vi "ecg_ncs_v1.vi"() -> ()   [LabVIEW 2016]
uses:
  <instrlib>/niUSRP/niUSRP Timestamp.ctl
  C:/Program Files/National Instruments/LabVIEW 2016/examples/Instrument IO/Serial/support/Serial - Settings.ctl
  State.ctl
  <vilib>/Instr/_visa.llb/VISA Configure Serial Port (Instr).vi
  <instrlib>/niUSRP/niUSRP Write Tx Data (2D CDB).vi
  <instrlib>/niUSRP/niUSRP Fetch Rx Data (2D CDB).vi
panel:
  out "error IO 2":errorcluster={"status"=FALSE, "code"=-1074118647, "source"=""}
  in  "Serial Settings":T1={"baud rate"=57600, "data bits"=8, "parity"=enum."None", "stop bits"=10, "flow control"=0} {"flow control" items=["None"=0, "XON/XOFF"=1, "RTS/CTS"=2, "DTR/DSR"=4]; "stop bits" items=["1.0"=10, "1.5"=15, "2.0"=20]; "data bits" min=5 max=8 step=1; "baud rate" items=["75"=75, "110"=110, "134"=134, "150"=150, "300"=300, "600"=600, "1200"=1200, "1800"=1800, "2400"=2400, "4800"=4800, "7200"=7200, "9600"=9600, "14400"=14400, "19200"=19200, "28800"=28800, "38400"=38400, "56000"=56000, "57600"=57600, "115200"=115200, "128000"=128000, "230400"=230400]}
  in  "VISA resource name":refnum<visa-resource-name>="bmd101"
  out "Packets Recieved":i32
  out "ECG":i16(graph)
  in  "byte count":u32=1
  in  "Stop 2":bool
  out "Coerced Rx IQ Rate":dbl
  in  "Sampling Rate":i32=500
  out "Gain":dbl=-15.0
  out "Bandwidth":dbl=56000000.0
  out "Coerced Carrier Frequency":dbl=2000000000.0 format="%#.17g"
  out "Coerced Tx IQ rate":dbl=1000000.0
  out "error IO":errorcluster={"status"=FALSE, "code"=-1074118647, "source"=""}
  in  "Rx Number of Samples":i32=20000
  in  "Tab Control 2":enum32{"NI-294x/295x", "NI-2900/2901"}(tab)=enum."NI-2900/2901"
  in  "Rx carrier frequency [Hz]":dbl=2000000000.0 format="%#_6p"
  in  "Tx carrier frequency [Hz]":dbl=1000000000.0 format="%#_6p"
  in  "Start Trigger Time":T2={"whole seconds"=1, "fractional seconds"=0.0}
  in  "Tab Control":T3(tab)
  out "NCS tag Amp":dbl[](graph)=[0.011967714738528729, 0.012021355192189592, 0.012015275039596582, 0.011969166030167903, 0.011958890166168242, 0.012007893820858737, 0.012022893722444085, 0.011978222225113794, 0.011969989939463181, 0.012003099640895068]
  out "NCS tag Phase":dbl[](graph)=[0.011967714738528729, 0.012021355192189592, 0.012015275039596582, 0.011969166030167903, 0.011958890166168242, 0.012007893820858737, 0.012022893722444085, 0.011978222225113794, 0.011969989939463181, 0.012003099640895068]
  out "Tag Amp":dbl[](graph)
  out "Tag Phase":dbl[](graph)
  out "Tx Waveform Graph":waveform(dbl)[](graph)
  in  "Stop":bool
  in  "Channel 0\nTone Amplitude":dbl=0.707 step=0.05 format="%#.6g"
  in  "Channel 0 \nTone Frequency":dbl=5000.0 format="%#_6p"
  in  "Tx Waveform Size":dbl=2000.0
  in  "Device Name":refnum<k15>="MyB200"
  in  "Tx Gain":dbl=28.0 format="%#_6f"
  in  "Tx IQ Rate":dbl=1000000.0 format="%#_6p"
  in  "Rx Gain":dbl=32.0 format="%#_6f"
  in  "Rx IQ Rate":dbl=1000000.0 format="%#_6p"
  # "Rx Settings"
  # "Tx Settings"
  # "Note that on the NI-2900 and NI-2901, both Rx channels share an LO and both Tx channels share an LO. However, on the NI-294x/295x devices, Rx and Tx of channel 0 share an LO and Rx and Tx of channel 1 share an LO."
  # "This Tx graph should always have end and start tied up since this is being sent in a loop continuously. Otherwise phase jumps will be noticed."
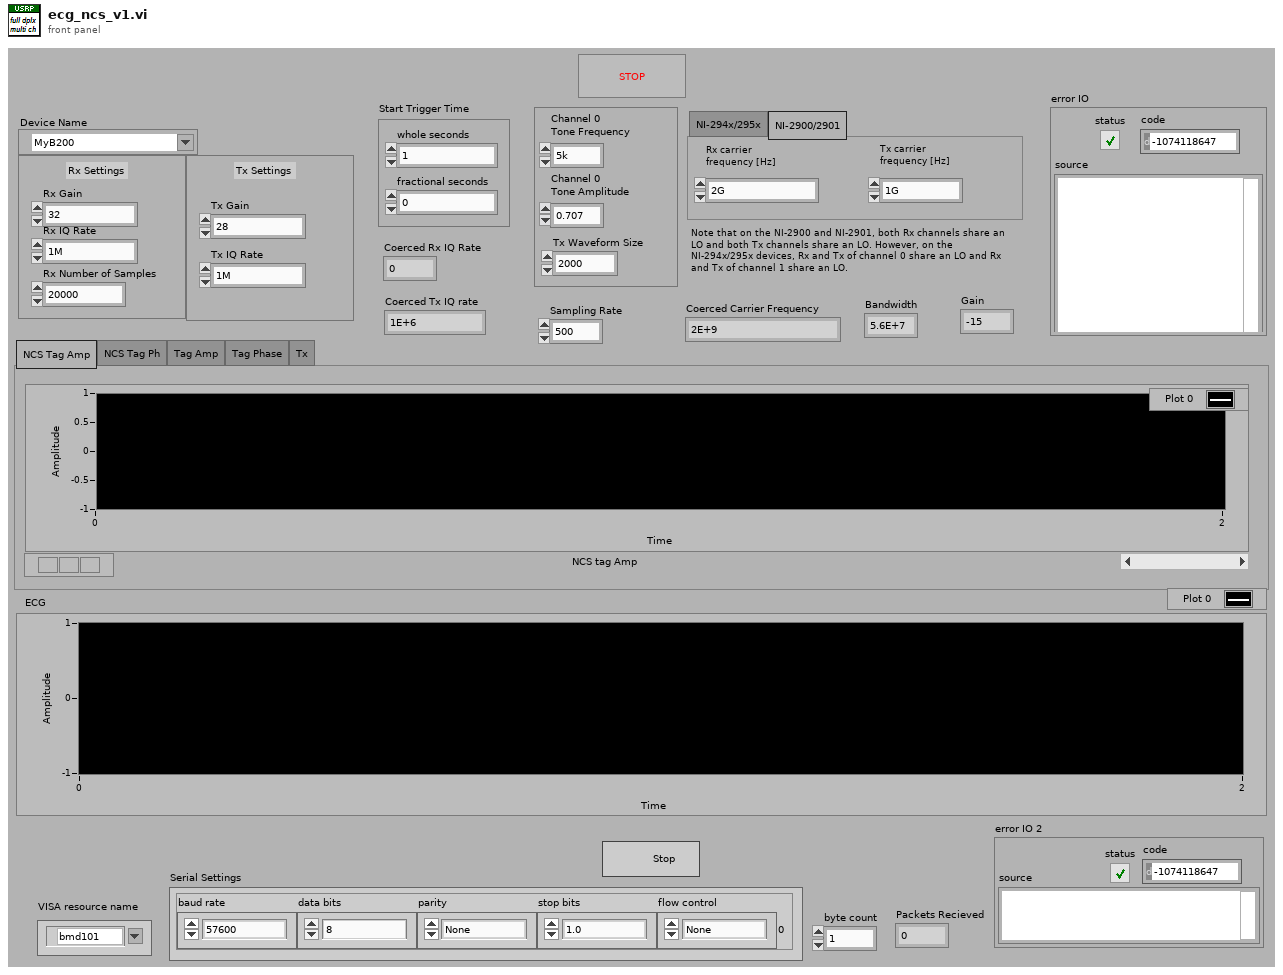
[diagram p1: front panel]
types:
  T1 = typedef "Serial - Settings.ctl" = cluster{"baud rate":u32, "data bits":u16, "parity":enum16{"None", "Odd", "Even", "Mark", "Space"}, "stop bits":u16, "flow control":u16}
  T2 = typedef "niUSRP Timestamp.ctl" = cluster{"whole seconds":u64, "fractional seconds":dbl}
  T3 = enum32{"NCS Tag Amp", "NCS Tag Ph", "Tag Amp", "Tag Phase", "Tx"}
  T4 = typedef "State.ctl" = enum16{"Initialize", "get byte", "check", "packet received", "packet approved"}
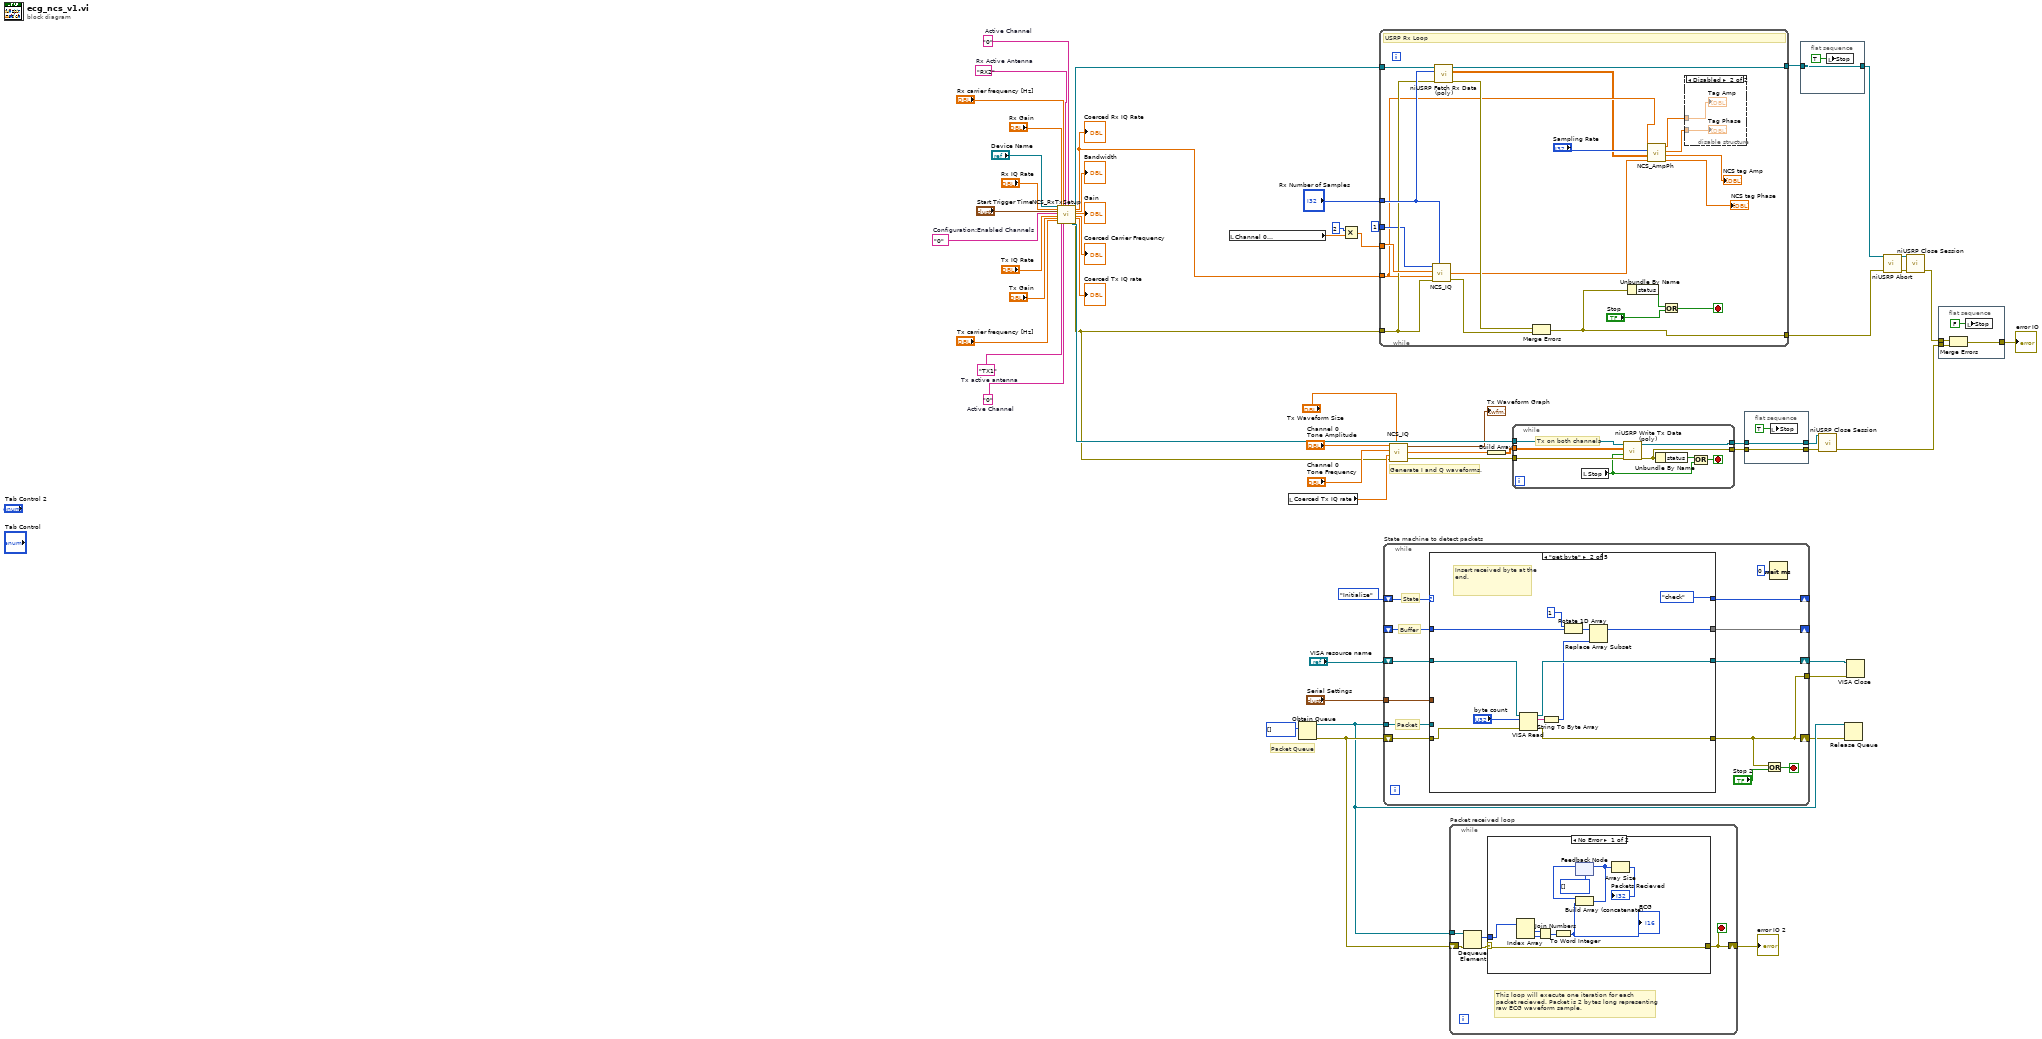
[diagram p0: block diagram]
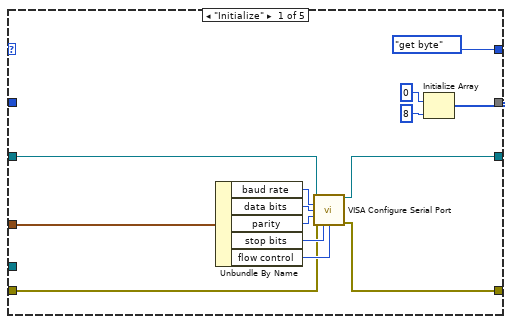
[diagram p3: hidden frame]
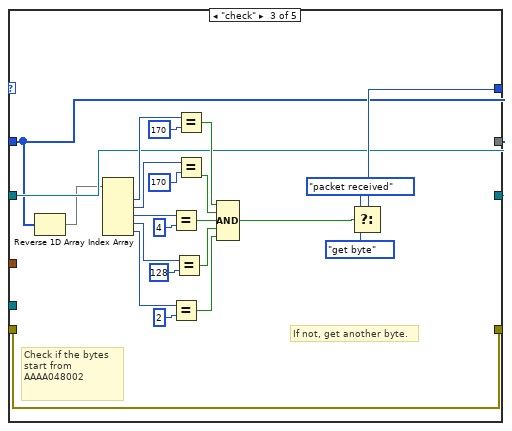
[diagram p4: hidden frame]
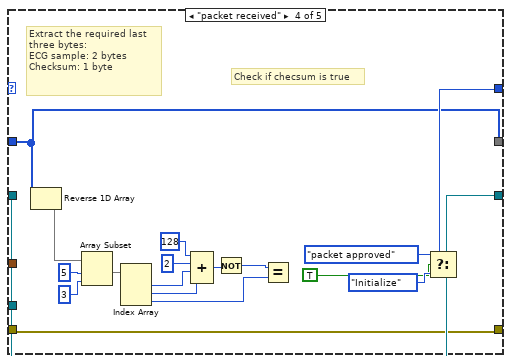
[diagram p5: hidden frame]
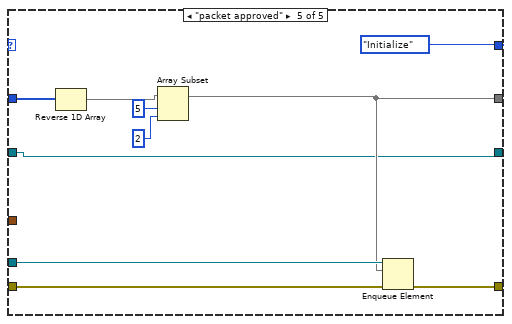
[diagram p6: hidden frame]
diagram:
  w12 = "0"  # Active Channel
  w13 = "0"  # Active Channel
  w48 = "RX2"  # Rx Active Antenna
  w44 = "TX1"  # Tx active antenna
  w30 = "0"  # Configuration:Enabled Channels
  # "Packet Queue"
  # "Generate I and Q waveforms."
  n1 = call "NCS_RxTxSetup.vi"("IVI Refnum in"="Device Name", "Rx IQ Rate"="Rx IQ Rate", "Start Trigger Time"="Start Trigger Time", "Configuration:Enabled Channels"=w30, "Tx IQ Rate"="Tx IQ Rate", "Tx Gain"="Tx Gain", "Tx carrier frequency [Hz]"="Tx carrier frequency [Hz]", "Rx Gain"="Rx Gain", "Tx active antenna"=w44, "Rx carrier frequency [Hz]"="Rx carrier frequency [Hz]", "Active Channel"=w12, "Rx Active Antenna"=w48, "Active Channel 2"=w13) -> ("session handle out"=w55:refnum<k15>, "IVI Refnum out"=w56:refnum<k15>, "Coerced Rx IQ Rate"=w11:dbl, "Bandwidth"=→"Bandwidth":dbl, "Gain"=→"Gain":dbl, "Carrier Frequency"=→"Coerced Carrier Frequency":dbl, "IQ Rate 2"=→"Coerced Tx IQ rate":dbl, "error out"=w23:errorcluster)  [unwired: 7 in]
  "Coerced Rx IQ Rate" <- w11
  n2 = local read "Channel 0 \nTone Frequency"() -> (w29:dbl)
  n3 = local read "Coerced Tx IQ rate"() -> (w24:dbl)
  n4 = Obtain Queue(element data type=u8[] []) -> (queue out=w7:refnum<queue>, error out=w8:errorcluster)  [unwired: 4 in, 1 out]
  n5 = Multiply(x=2, y=w29) -> (x*y=w28:dbl)
  n6 = while {
    tunnel: w56 -> [w76]
    tunnel: w23 -> [w68]
    tunnel: [w75] -> w40
    tunnel: "Rx Number of Samples" -> [w70]
    tunnel: w11 -> [w64]
    tunnel: [w65] -> w32
    tunnel: w28 -> [w69]
    tunnel: 1 -> [w66]
    stop <- w71 stop-if-true
    # "USRP Rx Loop"
    n7 = call "NCS_IQ.vi"("Tone Amplitude"=w66, "Waveform Size"=w70, "Tone Frequency"=w69, "Coerced IQ rate"=w64, "error in (no error)"=w68) -> ("IQ waveform array"=w61:cdb[], "error out"=w67:errorcluster)  [unwired: 1 in, 1 out]
    n8 = call-poly <instrlib>:"niUSRP Fetch Rx Data (poly).vi"("session handle"=w76, "number of samples"=w70, "error in (no error)"=w68) -> ("session handle out"=w75:refnum<k15>, "data"=w62:cdb[][], "error out"=w72:errorcluster)  [unwired: 9 in, 1 out]
    n9 = Merge Errors(w72, w67) -> (w65:errorcluster)
    n10 = Unbundle By Name(w65) -> ("status"=w74:bool)
    n11 = call "NCS_AmpPh.vi"("IQ"=w61, "data"=w62, "Sampling Rate"="Sampling Rate", "Coerced Rx IQ Rate"=w64) -> ("Phase DownSampled"=→"NCS tag Phase":dbl[], "Amp DownSampled"=→"NCS tag Amp":dbl[], "Unfiltered Phase"=w59:dbl[], "Unfiltered Amplitude"=w60:dbl[])  [unwired: 4 in]
    n12 = Or(x=w74, y="Stop") -> (x .or. y?=w71:bool)
    n13 = disable-structure shown="Disabled" {
      disable-tunnel: w60 -> [_ w78]
      disable-tunnel: w59 -> [_ w77]
      frame Enabled {
      }
      frame Disabled {
        "Tag Amp" <- w78
        "Tag Phase" <- w77
      }
    }
  }
  n14 = while "State machine to detect packets" {
    shift-right: [w82] -> w2
    shift-left: w8 -> [w88]
    shift-right: [w91] -> _
    shift-left: State."Initialize" ("State") -> [w90]
    shift-right: [w87] -> _
    shift-left: _ -> [w89]
    tunnel: w7 -> [w86]
    shift-right: [w85] -> w3
    shift-left: "VISA resource name" -> [w84]
    tunnel: "Serial Settings" -> [w83]
    tunnel: [w82] -> w1
    stop <- w80 stop-if-true
    # "State"
    # "Buffer"
    # "Packet"
    n15 = case shown="\"get byte\"" w90 {
      tunnel: [w102 w115 w119 w142 w162] -> w87
      tunnel: [State."get byte" ("State") State."check" ("f") w139 w148 State."Initialize" ("State")] -> w91
      tunnel: w89 -> [_ w107 w119 w142 w160]
      tunnel: w88 -> [w96 w111 w140 w149 w164]
      tunnel: [w95 w110 w140 w149 w163] -> w82
      tunnel: w86 -> [_ _ _ _ w165]
      tunnel: [w94 w113 w120 w156 w161] -> w85
      tunnel: w84 -> [w93 w114 w120 w156 w161]
      tunnel: w83 -> [w92 _ _ _ _]
      frame "Initialize" {
        n16 = Unbundle By Name(w92) -> ("baud rate"=w101:u32, "data bits"=w100:u16, "parity"=w99:enum16{"None", "Odd", "Even", "Mark", "Space"}, "stop bits"=w98:u16, "flow control"=w97:u16)
        n17 = call-poly "VISA Configure Serial Port"("VISA resource name"=w93, "baud rate (9600)"=w101, "data bits (8)"=w100, "parity (0:none)"=w99, "error in (no error)"=w96, "stop bits (10: 1 bit)"=w98, "flow control (0:none)"=w97) -> ("VISA resource name out"=w94:refnum<visa-resource-name>, "error out"=w95:errorcluster)  [unwired: 3 in, 4 out]
        n18 = Initialize Array(u8 0, 8 ("dimension size")) -> (w102:u8[])
      }
      frame "get byte" {
        # "Insert received byte at the end."
        n19 = VISA Read(VISA resource name=w114, byte count="byte count", error in (no error)=w111) -> (VISA resource name out=w113:refnum<visa-resource-name>, read buffer=w109:string, error out=w110:errorcluster)  [unwired: 1 out]
        n20 = String To Byte Array(string=w109) -> (unsigned byte array=w108:u8[])
        n21 = Rotate 1D Array(1:w107, 2:1) -> (0:w116:u8[])
        n22 = Replace Array Subset(array=w116, new element=w108) -> (w115:u8[])  [unwired: 1 in]
      }
      frame "check" {
        # "If not, get another byte."
        # "Check if the bytes start from AAAA048002"
        n23 = Reverse 1D Array(array=w119) -> (reversed array=w118:u8[])
        n24 = Index Array(array=w118) -> (element #1=w126:u8, element #2=w125:u8, element #3=w124:u8, element #4=w123:u8, element #5=w122:u8)  [unwired: 5 in]
        n25 = Equal?(x=w124, y=u8 4 ("element")) -> (x = y?=w129:bool)
        n26 = Equal?(x=w122, y=u8 2 ("element")) -> (x = y?=w127:bool)
        n27 = Equal?(x=w123, y=u8 128 ("element")) -> (x = y?=w128:bool)
        n28 = Equal?(x=w126, y=u8 170 ("element")) -> (x = y?=w131:bool)
        n29 = Equal?(x=w125, y=u8 170 ("element")) -> (x = y?=w130:bool)
        n30 = Compound Arithmetic op=AND(w131, w130, w129, w128, w127) -> (w121:bool)
        n31 = Select(t=State."packet received" ("f"), s=w121, f=State."get byte") -> (s? t:f=w139:T4)
      }
      frame "packet received" {
        # "Check if checsum is true"
        # "Extract the required last three bytes: \nECG sample: 2 bytes\nChecksum: 1 byte"
        n32 = Reverse 1D Array(array=w142) -> (reversed array=w141:u8[])
        n33 = Array Subset(array=w141, index=5, length=3 ("index")) -> (w155:u8[])
        n34 = Index Array(array=w155) -> (element #1=w150:u8, element #2=w151:u8, element #3=w152:u8)  [unwired: 3 in]
        n35 = Compound Arithmetic op=ADD(u8 128 ("element"), u8 2 ("element"), w150, w151) -> (w145:u8)
        n36 = Not(x=w145) -> (.not. x?=w144:u8)
        n37 = Equal?(x=w144, y=w152) -> ()  [unwired: 1 out]
        n38 = Select(t=State."packet approved" ("State"), s=TRUE, f=State."Initialize" ("State")) -> (s? t:f=w148:T4)
      }
      frame "packet approved" {
        n39 = Reverse 1D Array(array=w160) -> (reversed array=w159:u8[])
        n40 = Array Subset(array=w159, index=5, length=2 ("index")) -> (w162:u8[])
        n41 = Enqueue Element(queue=w165, element=w162, error in (no error)=w164) -> (error out=w163:errorcluster)  [unwired: 1 in, 2 out]
      }
    }
    n42 = Or(x=w82, y="Stop 2") -> (x .or. y?=w80:bool)
    n43 = Wait (ms)(milliseconds to wait=u32 0) -> ()  [unwired: 1 out]
  }
  n44 = call "NCS_IQ.vi"("Tone Amplitude"="Channel 0\nTone Amplitude", "Waveform Size"="Tx Waveform Size", "Tone Frequency"="Channel 0 \nTone Frequency", "Coerced IQ rate"=w24, "error in (no error)"=w23) -> ("IQ waveform"=→"Tx Waveform Graph":waveform(dbl)[], "IQ waveform array"=w21:cdb[], "error out"=w22:errorcluster)  [unwired: 1 in]
  n45 = while "Packet received loop" {
    shift-right: [w169] -> w4
    shift-left: w8 -> [w173]
    tunnel: w7 -> [w172]
    stop <- w169 stop-if-true
    # "This loop will execute one iteration for each\npacket recieved. Packet is 2 bytes long representing \nraw ECG waveform sample."
    n46 = Dequeue Element(queue=w172, error in (no error)=w173) -> (element=w171:u8[], error out=w170:errorcluster)  [unwired: 1 in, 2 out]
    n47 = case shown="No Error" w170 {
      selector: w170 -> [w183 w184]
      tunnel: w171 -> [w182 _]
      tunnel: [w183 w184] -> w169
      frame No Error {
        n48 = Index Array(array=w182) -> (element #1=w181:u8, element #2=w180:u8)  [unwired: 2 in]
        n49 = Join Numbers(hi=w181, lo=w180) -> ((hi.lo)=w179:u16)
        n50 = To Word Integer(number=w179) -> (16bit integer=w174:i16)
        "ECG" <- w174
        n51 = feedback #1(i32[] []) -> (w177:i32[])
        n52 = Build Array (concatenate)(w177, w174) -> (w176:i32[])
        n53 = feedback-in #1(w176) -> ()
        n54 = Array Size(array=w176) -> (size(s)=→"Packets Recieved":i32)
      }
      frame Error {
      }
    }
  }
  "error IO 2" <- w4
  n55 = Build Array(w21) -> (w52:cdb[][])
  n56 = while {
    tunnel: w55 -> [w192]
    tunnel: w22 -> [w191]
    tunnel: [w189] -> w43
    tunnel: [w187] -> w38
    tunnel: w52 -> [w185]
    stop <- w188 stop-if-true
    # "Tx on both channels"
    n57 = local read "Stop"() -> (w186:bool)
    n58 = call-poly <instrlib>:"niUSRP Write Tx Data (poly).vi"("session handle"=w192, "data"=w185, "end of data?"=w186, "error in (no error)"=w191) -> ("session handle out"=w187:refnum<k15>, "error out"=w189:errorcluster)  [unwired: 10 in]
    n59 = Unbundle By Name(w189) -> ("status"=w190:bool)
    n60 = Compound Arithmetic op=OR(w190, w186) -> (w188:bool)
  }
  n61 = flat-sequence {
    tunnel: [w194] -> w42
    tunnel: w43 -> [w194]
    tunnel: [w193] -> w39
    tunnel: w38 -> [w193]
    frame #0 {
      n62 = local write "Stop"(TRUE ("STOP")) -> ()
    }
  }
  n63 = flat-sequence {
    tunnel: [w196] -> w41
    tunnel: w40 -> [w196]
    frame #0 {
      n64 = local write "Stop"(TRUE ("STOP")) -> ()
    }
  }
  n65 = call <instrlib>:"niUSRP Close Session.vi"("session handle"=w39, "error in (no error)"=w42) -> ("error out"=w37:errorcluster)  [unwired: 13 in]
  n66 = Release Queue(queue=w7, error in (no error)=w2) -> ()  [unwired: 1 in, 3 out]
  n67 = VISA Close(VISA resource name=w3, error in (no error)=w1) -> ()  [unwired: 1 out]
  n68 = call <instrlib>:"niUSRP Abort.vi"("session handle"=w41, "error in (no error)"=w32) -> ("session handle out"=w54:refnum<k15>, "error out"=w53:errorcluster)  [unwired: 12 in]
  n69 = call <instrlib>:"niUSRP Close Session.vi"("session handle"=w54, "error in (no error)"=w53) -> ("error out"=w34:errorcluster)  [unwired: 13 in]
  n70 = flat-sequence {
    tunnel: w37 -> [w200]
    tunnel: [w199] -> w35
    tunnel: w34 -> [w198]
    frame #0 {
      n71 = Merge Errors(w198, w200) -> (w199:errorcluster)
      n72 = local write "Stop"(FALSE ("STOP")) -> ()
    }
  }
  "error IO" <- w35
